vi "ZMC Get In All.vi"(7 "pistate":u32, 8 "error in (no error)":errorcluster caption="错误输入（无错误）", 9 "inumend":u16, 10 "inumfirst":u16, 11 "handle":u32) -> (0 "error out":errorcluster caption="错误输出", 2 "function return":i32, 3 "handle out":u32, 5 "pistate out":u32)   [LabVIEW 2019, in "zauxdll.lvlib"]
doc: "int32 __stdcall ZMC_GetInAll(ZMC_HANDLE handle, uint16 inumfirst,uint16 inumend, uint32* pistate);"
uses:
  zauxdll.lvlib
  zmotion.dll
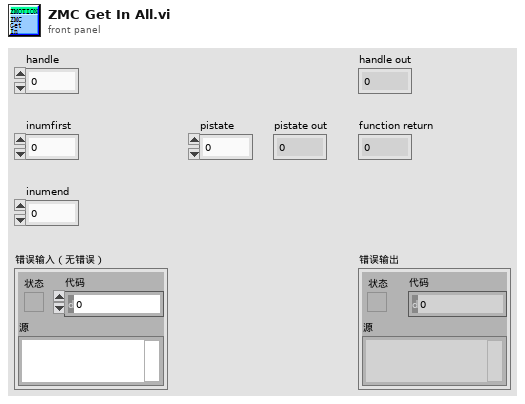
[diagram p1: front panel]
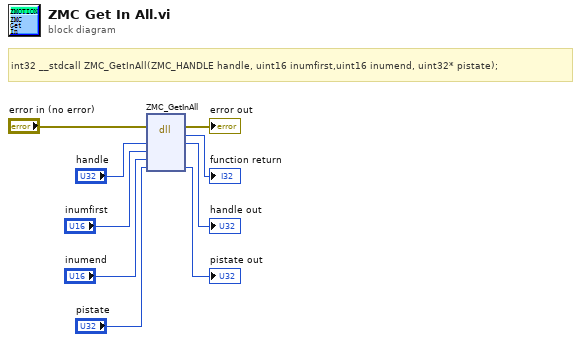
[diagram p0: block diagram]
diagram:
  # "int32 __stdcall ZMC_GetInAll(ZMC_HANDLE handle, uint16 inumfirst,uint16 inumend, uint32* pistate);"
  n1 = dll-call lib="C:/Users/VIC/Desktop/Standar Program/System/LLB/zmotion/zaux/zmotion.*" fn="ZMC_GetInAll"(error in="error in (no error)", "handle"="handle", "inumfirst"="inumfirst", "inumend"="inumend", "pistate"="pistate") -> (error out=→"error out":errorcluster, →"function return":i32, "handle"=→"handle out":u32, "pistate"=→"pistate out":u32)  [unwired: 4 in, 1 out]
